vi "Autofocus Start.vi"(8 "error in (no error)":errorcluster, 11 "Stage Controller in":refnum<class "Stage Controller.lvclass">) -> (0 "error out":errorcluster, 3 "Stage Controller out":refnum<class "Stage Controller.lvclass">)   [LabVIEW 2023, in "Stage Controller.lvlib" / "Stage Controller.lvclass"]
uses:
  Stage Controller.lvclass
  Stage Controller.lvclass/Stage Controller.ctl
  Stage Axis.ctl
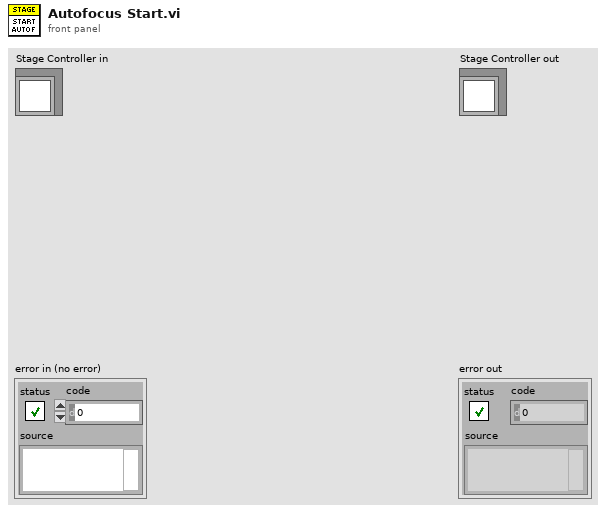
[diagram p1: front panel]
types:
  T1 = typedef "Stage Controller.lvlib/Stage Controller.lvclass/Stage Axis.ctl" = enum16{"unspecified", "X", "Y", "Z"}
  T2 = typedef "Stage Position.ctl" = cluster{"X (mm)":dbl, "Y (mm)":dbl, "Z (mm)":dbl}
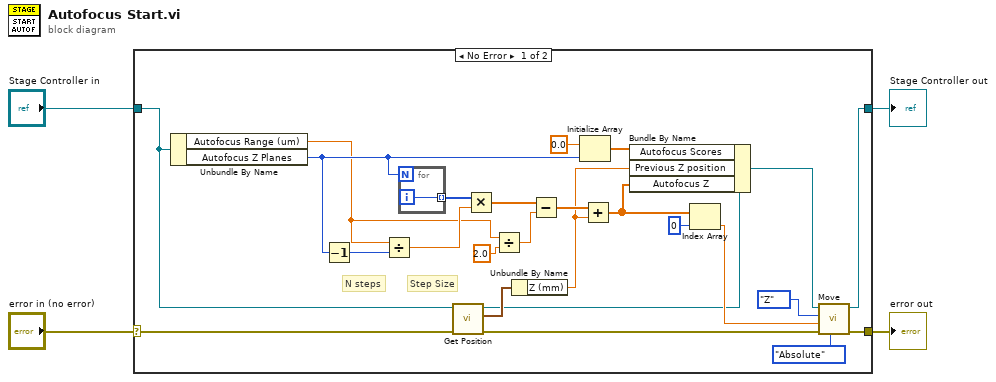
[diagram p0: block diagram]
diagram:
  n1 = case shown="No Error" "error in (no error)" {
    selector: "error in (no error)" -> [w13 w32]
    tunnel: [w7 w32] -> w3
    tunnel: [w8 w31] -> w1
    tunnel: "Stage Controller in" -> [w14 w31]
    frame No Error {
      # "Step Size"
      # "N steps"
      n2 = Unbundle By Name(w14) -> ("Autofocus Range (um)"=w18:dbl, "Autofocus Z Planes"=w24:i32)
      n3 = Decrement(x=w24) -> (x-1=w26:i32)
      n4 = Divide(x=w18, y=w26) -> (x/y=w27:dbl)
      n5 = for {
        N: w24 -> [_]
        tunnel: [w30] -> w23 mode=indexing
        i -> [w30]
      }
      n6 = call-dynamic "Get Position.vi"("error in (no error)"=w13, "Stage Controller in"=w14) -> ("error out"=w11:errorcluster, "Stage Position"=w16:T2, "Stage Controller out"=w10:refnum<class "Stage Controller.lvclass">)  [unwired: 6 in, 1 out]
      n7 = Multiply(x=w23, y=w27) -> (x*y=w20:dbl[])
      n8 = Divide(x=w18, y=2.0) -> (x/y=w22:dbl)
      n9 = Unbundle By Name(w16) -> ("Z (mm)"=w15:dbl)
      n10 = Subtract(x=w20, y=w22) -> (x-y=w19:dbl[])
      n11 = Initialize Array(0.0 ("element"), w24) -> (w29:dbl[])
      n12 = Add(x=w19, y=w15) -> (x+y=w17:dbl[])
      n13 = Bundle By Name(cluster=w10, "Autofocus Scores"=w29, "Previous Z position"=w15, "Autofocus Z"=w17) -> (w9:refnum<class "Stage Controller.lvclass">)
      n14 = Index Array(array=w17, index=0) -> (element=w12:dbl)
      n15 = call-dynamic "Move.vi"("Mode"=enum16{"Relative", "Absolute"}."Absolute", "error in (no error)"=w11, "Value (mm)"=w12, "Axis"=Stage_Axis."Z", "Stage Controller in"=w9) -> ("error out"=w7:errorcluster, "Stage Controller out"=w8:refnum<class "Stage Controller.lvclass">)  [unwired: 5 in]
    }
    frame Error {
    }
  }
  "error out" <- w3
  "Stage Controller out" <- w1
